vi "getDataPath.vi"(8 "error in (no error)":errorcluster) -> (0 "error out":errorcluster, 2 "DataPath":path)   [LabVIEW 2011]
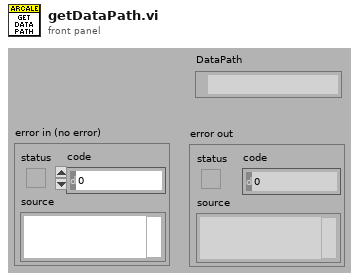
[diagram p1: front panel]
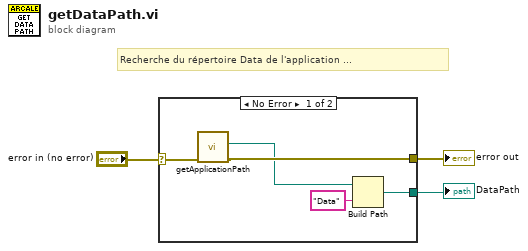
[diagram p0: block diagram]
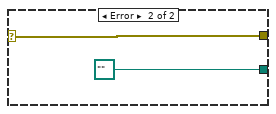
[diagram p2: hidden frame]
diagram:
  # "Recherche du répertoire Data de l'application ..."
  n1 = case shown="No Error" "error in (no error)" {
    selector: "error in (no error)" -> [w6 w9]
    tunnel: [w7 path "" ("appended path")] -> w3
    tunnel: [w5 w9] -> w1
    frame No Error {
      n2 = call "getApplicationPath.vi"("error in (no error)"=w6) -> ("error out"=w5:errorcluster, "ApplicationPath"=w4:path)  [unwired: 9 in]
      n3 = Build Path(base path=w4, name or relative path="Data") -> (appended path=w7:path)
    }
    frame Error {
    }
  }
  "error out" <- w1
  "DataPath" <- w3
